vi "Color_Project.vi"() -> ()   [LabVIEW 2013]
uses:
  leitura de dados txt control.ctl
panel:
  out "Color Box":u32(colorbox)
  out "RGB":dbl[](array[numeric])
  in  "RGBStandards":string(combo)
  out "XYZ":dbl[](array[numeric])
  out "L*a*b*":dbl[](array[numeric])
  out "r1":dbl[](array[numeric])
  out "Reflectance2":string[][](array[string])
  out "teste":i32[](array[numeric])
  out "IL Table":string[][](array[string])
  out "ILCols":i32
  out "ILRows":i32
  out "Selected illuminant":dbl[](array[numeric])
  out "Reflectance":i32[](array[numeric])
  out "Is CMF selected?":bool
  out "Is illuminant selected?":bool
  out "Intepoled iluminants":dbl[][](array[numeric])
  out "Selected\nCMF":dbl[][](array[numeric])
  out "cmf Index":dbl
  out "CMFCols":i32
  out "CMFRows":i32
  out "CMF Table":string[][](array[string])
  in  "Color Matching Function":string(combo)
  out "Illuminant Graph":T1(graph)
  out "LambdaInterval":dbl[](array[numeric])
  out "NeedInterpolation?":bool
  out "Selected illuminant index":dbl
  in  "Select Illuminant":T2
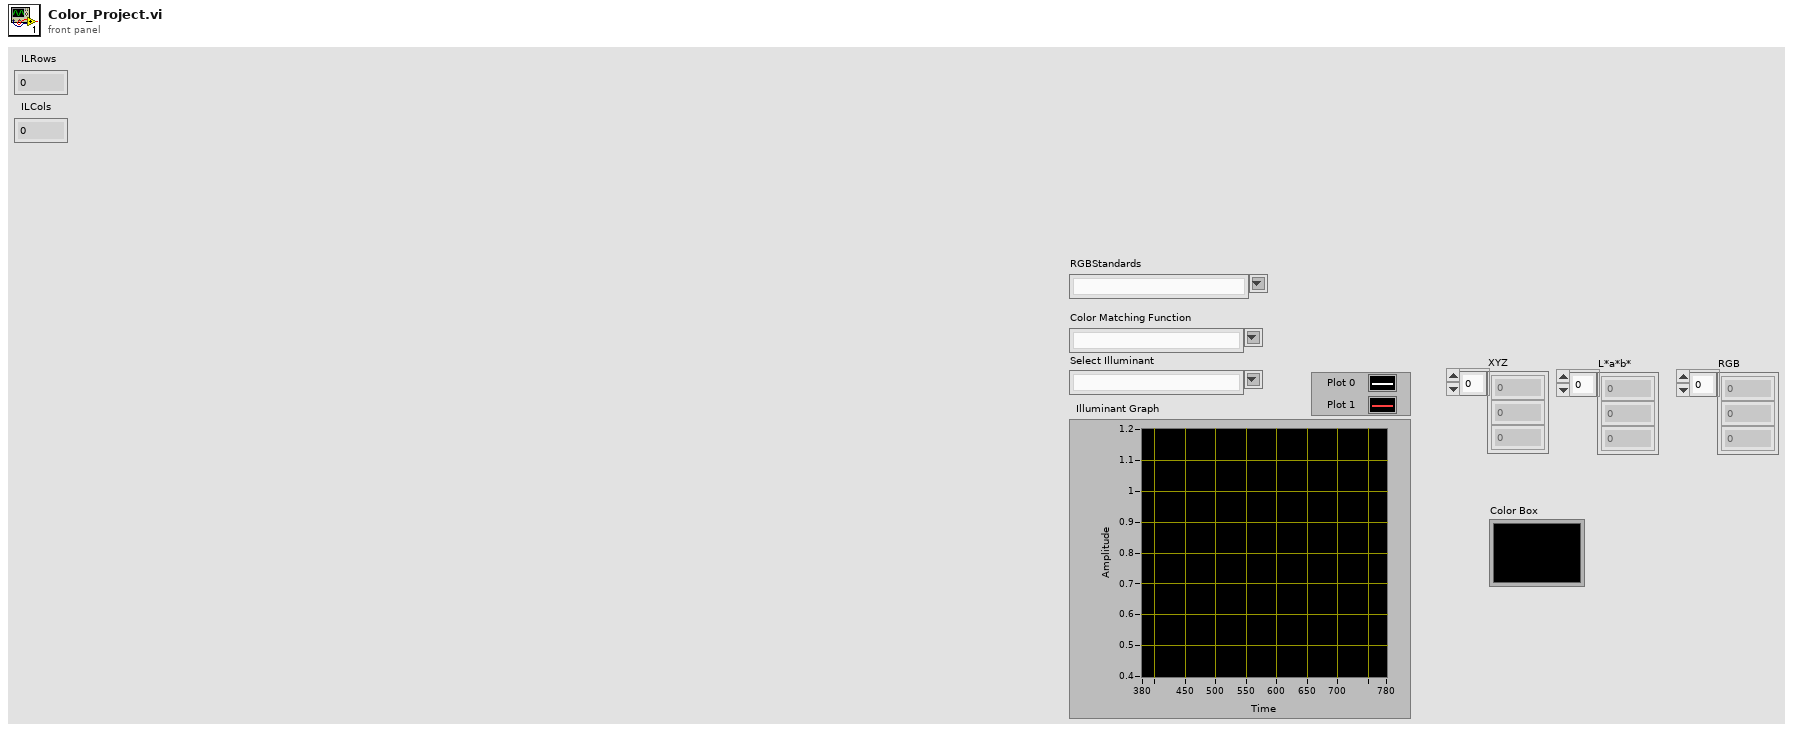
[diagram p1: front panel]
types:
  T1 = cluster{"GammaInterval":dbl[], "Interpolated":dbl[]}[]
  T2 = typedef "leitura de dados txt control.ctl" = string
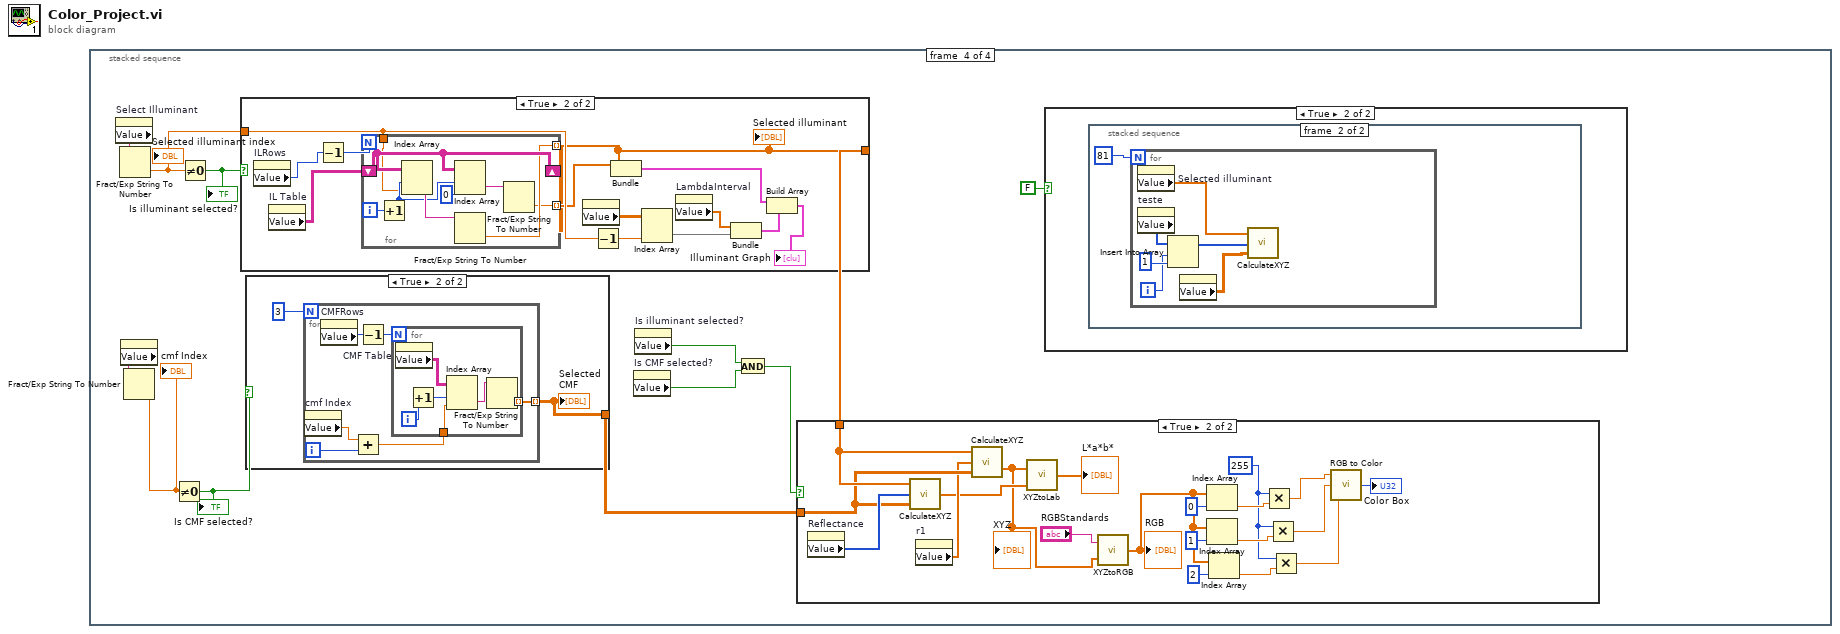
[diagram p0: block diagram]
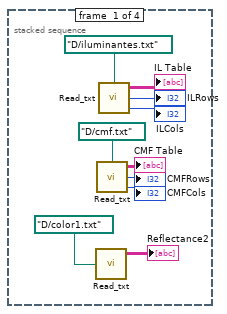
[diagram p2: hidden frame]
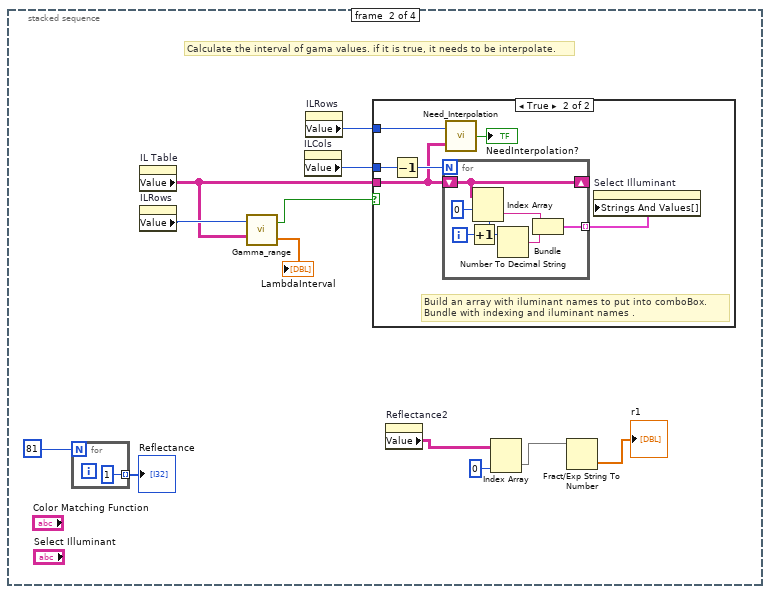
[diagram p3: hidden frame]
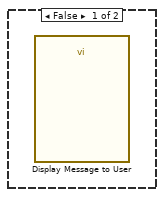
[diagram p4: hidden frame]
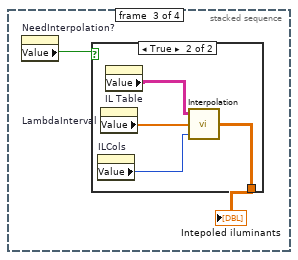
[diagram p5: hidden frame]
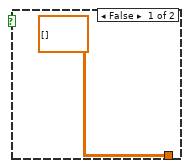
[diagram p6: hidden frame]
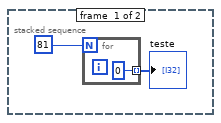
[diagram p8: hidden frame]
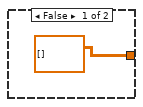
[diagram p10: hidden frame]
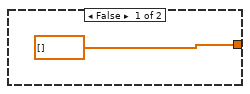
[diagram p11: hidden frame]
diagram:
  n1 = stacked-sequence {
    frame #0 {
      n2 = call "Read_txt.vi"("file path (dialog if empty)"=path "D:/color1.txt") -> ("Elements"=→"Reflectance2":string[][])  [unwired: 2 out]
      n3 = call "Read_txt.vi"("file path (dialog if empty)"=path "D:/cmf.txt") -> ("Elements"=→"CMF Table":string[][], "Rows"=→"CMFRows":i32, "Cols"=→"CMFCols":i32)
      n4 = call "Read_txt.vi"("file path (dialog if empty)"=path "D:/iluminantes.txt") -> ("Elements"=→"IL Table":string[][], "Rows"=→"ILRows":i32, "Cols"=→"ILCols":i32)
    }
    frame #1 {
      # "Calculate the interval of gama values. if it is true, it needs to be interpolate."
      n5 = for {
        N: 81 -> [_]
        tunnel: [1] -> w21 mode=indexing
      }
      "Reflectance" <- w21
      n6 = property on="IL Table" class="Arr (strict)"() -> ("Value"=w18:string[][])  [unwired: 2 in, 2 out]
      n7 = property on="ILRows" class="DigNum (strict)"() -> ("Value"=w19:i32)  [unwired: 2 in, 2 out]
      n8 = call "Gamma_range.vi"("Illuminant Table"=w18, "NumberOfRows"=w19) -> ("GammaInterval"=→"LambdaInterval":dbl[], "In range?"=w15:bool)
      n9 = property on="ILCols" class="DigNum (strict)"() -> ("Value"=w17:i32)  [unwired: 2 in, 2 out]
      n10 = property on="ILRows" class="DigNum (strict)"() -> ("Value"=w16:i32)  [unwired: 2 in, 2 out]
      n11 = case shown="True" w15 {
        tunnel: w18 -> [_ w24]
        tunnel: w17 -> [_ w25]
        tunnel: w16 -> [_ w23]
        frame False {
          n12 = call "Display Message to User"() -> ()  [unwired: 10 in, 2 out]
        }
        frame True {
          # "Build an array with iluminant names to put into comboBox.\nBundle with indexing and iluminant names ."
          n13 = Decrement(x=w25) -> (x-1=w27:i32)
          n14 = for {
            N: w27 -> [_]
            shift-right: [w33] -> _
            shift-left: w24 -> [w33]
            tunnel: [w29] -> w26 mode=indexing
            i -> [w35]
            n15 = Increment(x=w35) -> (x+1=w32:i32)
            n16 = Index Array(array=w33, index (row)=0, index (col)=w32) -> (element=w30:string)
            n17 = Number To Decimal String(number=w32) -> (decimal integer string=w31:string)  [unwired: 1 in]
            n18 = Bundle("String"=w30, w31) -> (w29:cluster{"String":string, string})  [unwired: 1 in]
          }
          n19 = call "Need_Interpolation.vi"("Matrix with txt"=w24, "Number of Rows"=w23) -> ("isNotFive?"=→"NeedInterpolation?":bool)
          n20 = property on="Select Illuminant" class="CmbBox (strict)"("Strings And Values[]"=w26) -> ()  [unwired: 2 in, 2 out]
        }
      }
      n21 = property on="Reflectance2" class="Arr (strict)"() -> ("Value"=w14:string[][])  [unwired: 2 in, 2 out]
      n22 = Index Array(array=w14, index (col)=0 ("disabled index (col)")) -> (element=w12:string[])  [unwired: 1 in]
      n23 = Fract/Exp String To Number(string=w12) -> (number=→"r1":dbl[])  [unwired: 3 in, 1 out]
    }
    frame #2 {
      n24 = property on="NeedInterpolation?" class="Bool (strict)"() -> ("Value"=w38:bool)  [unwired: 2 in, 2 out]
      n25 = case shown="True" w38 {
        tunnel: [dbl[][] [] w42] -> w37
        frame False {
        }
        frame True {
          n26 = property on="ILCols" class="DigNum (strict)"() -> ("Value"=w40:i32)  [unwired: 2 in, 2 out]
          n27 = property on="LambdaInterval" class="Arr (strict)"() -> ("Value"=w43:dbl[])  [unwired: 2 in, 2 out]
          n28 = property on="IL Table" class="Arr (strict)"() -> ("Value"=w41:string[][])  [unwired: 2 in, 2 out]
          n29 = call "Interpolation.vi"("Number of Columns"=w40, "Lambda Interval"=w43, "Illuminants"=w41) -> ("Interpolated"=w42:dbl[][])
        }
      }
      "Intepoled iluminants" <- w37
    }
    frame #3 {
      n30 = property on="Select Illuminant" class="CmbBox (strict)"() -> ("Value"=w51:T2)  [unwired: 2 in, 2 out]
      n31 = Fract/Exp String To Number(string=w51) -> (number=w50:dbl)  [unwired: 3 in, 1 out]
      "Selected illuminant index" <- w50
      n32 = property on="Color Matching Function" class="CmbBox"() -> ("Value"=w53:string)  [unwired: 2 in, 2 out]
      n33 = Fract/Exp String To Number(string=w53) -> (number=w54:dbl)  [unwired: 3 in, 1 out]
      "cmf Index" <- w54
      n34 = Not Equal To 0?(x=w54) -> (x != 0?=w52:bool)
      "Is CMF selected?" <- w52
      n35 = Not Equal To 0?(x=w50) -> (x != 0?=w55:bool)
      "Is illuminant selected?" <- w55
      n36 = case shown="True" w55 {
        tunnel: w50 -> [_ w110]
        tunnel: [dbl[] [] w104] -> w45
        frame False {
        }
        frame True {
          n37 = property on="ILRows" class="DigNum (strict)"() -> ("Value"=w103:i32)  [unwired: 2 in, 2 out]
          n38 = property on="IL Table" class="Arr (strict)"() -> ("Value"=w102:string[][])  [unwired: 2 in, 2 out]
          n39 = Decrement(x=w103) -> (x-1=w114:i32)
          n40 = for {
            N: w114 -> [_]
            shift-right: [w122] -> _
            shift-left: w102 -> [w122]
            tunnel: w110 -> [w115]
            tunnel: [w117] -> w104 mode=indexing
            tunnel: [w116] -> w106 mode=indexing
            i -> [w123]
            n41 = Increment(x=w123) -> (x+1=w118:i32)
            n42 = Index Array(array=w122, index (row)=w118, index (col)=w115) -> (element=w119:string)
            n43 = Index Array(array=w122, index (row)=w118, index (col)=0 ("disabled index (col)")) -> (element=w120:string)
            n44 = Fract/Exp String To Number(string=w119) -> (number=w117:dbl)  [unwired: 3 in, 1 out]
            n45 = Fract/Exp String To Number(string=w120) -> (number=w116:dbl)  [unwired: 3 in, 1 out]
          }
          "Selected illuminant" <- w104
          n46 = property on="Intepoled iluminants" class="Arr (strict)"() -> ("Value"=w108:dbl[][])  [unwired: 2 in, 2 out]
          n47 = Decrement(x=w110) -> (x-1=w109:dbl)
          n48 = Bundle(w106, w104) -> (w111:cluster{dbl[], dbl[]})  [unwired: 1 in]
          n49 = Index Array(array=w108, index (col)=w109) -> (element=w105:dbl[])  [unwired: 1 in]
          n50 = property on="LambdaInterval" class="Arr (strict)"() -> ("Value"=w107:dbl[])  [unwired: 2 in, 2 out]
          n51 = Bundle("Value"=w107, "Value"=w105) -> (w112:cluster{"Value":dbl[], "Value":dbl[]})  [unwired: 1 in]
          n52 = Build Array(w111, w112) -> (→"Illuminant Graph":cluster{"Value":dbl[], "Value":dbl[]}[])
        }
      }
      n53 = case shown="True" w52 {
        tunnel: [dbl[][] [] w87] -> w46
        frame False {
        }
        frame True {
          n54 = for {
            N: 3 -> [_]
            tunnel: [w91] -> w87 mode=indexing
            i -> [w93]
            n55 = property on="cmf Index" class="DigNum (strict)"() -> ("Value"=w94:dbl)  [unwired: 2 in, 2 out]
            n56 = property on="CMFRows" class="DigNum (strict)"() -> ("Value"=w90:i32)  [unwired: 2 in, 2 out]
            n57 = Add(x=w94, y=w93) -> (x+y=w92:dbl)
            n58 = Decrement(x=w90) -> (x-1=w89:i32)
            n59 = for {
              N: w89 -> [_]
              tunnel: w92 -> [w99]
              tunnel: [w95] -> w91 mode=indexing
              i -> [w98]
              n60 = property on="CMF Table" class="Arr (strict)"() -> ("Value"=w100:string[][])  [unwired: 2 in, 2 out]
              n61 = Increment(x=w98) -> (x+1=w97:i32)
              n62 = Index Array(array=w100, index (row)=w97, index (col)=w99) -> (element=w96:string)
              n63 = Fract/Exp String To Number(string=w96) -> (number=w95:dbl)  [unwired: 3 in, 1 out]
            }
          }
          "Selected\nCMF" <- w87
        }
      }
      n64 = property on="Is CMF selected?" class="Bool (strict)"() -> ("Value"=w48:bool)  [unwired: 2 in, 2 out]
      n65 = property on="Is illuminant selected?" class="Bool (strict)"() -> ("Value"=w49:bool)  [unwired: 2 in, 2 out]
      n66 = And(x=w49, y=w48) -> (x .and. y?=w47:bool)
      n67 = case shown="True" w47 {
        tunnel: w45 -> [_ w84]
        tunnel: w46 -> [_ w83]
        frame False {
        }
        frame True {
          w69 = 255
          n68 = property on="Reflectance" class="Arr (strict)"() -> ("Value"=w85:i32[])  [unwired: 2 in, 2 out]
          n69 = call "CalculateXYZ.vi"("CMF"=w83, "Reflectance"=w85, "Illuminant"=w84) -> ("XYZ"=w81:dbl[])
          n70 = property on="r1" class="Arr (strict)"() -> ("Value"=w82:dbl[])  [unwired: 2 in, 2 out]
          n71 = call "CalculateXYZ.vi"("CMF"=w83, "Reflectance"=w82, "Illuminant"=w84) -> ("XYZ"=w79:dbl[])
          "XYZ" <- w79
          n72 = call "XYZtoLab.vi"("XrYrZr"=w81, "XYZ"=w79) -> ("L*a*b*"=→"L*a*b*":dbl[])
          n73 = call "XYZtoRGB.vi"("XYZ"=w79, "RGBStandards"="RGBStandards") -> ("RGB"=w76:dbl[])
          "RGB" <- w76
          n74 = Index Array(array=w76, index=0) -> (element=w72:dbl)
          n75 = Index Array(array=w76, index=1) -> (element=w70:dbl)
          n76 = Index Array(array=w76, index=2) -> (element=w71:dbl)
          n77 = Multiply(x=w69, y=w72) -> (x*y=w68:dbl)
          n78 = Multiply(x=w69, y=w70) -> (x*y=w67:dbl)
          n79 = Multiply(x=w69, y=w71) -> (x*y=w66:dbl)
          n80 = call <vilib>:"RGB to Color.vi"("B"=w66, "G"=w67, "R"=w68) -> ("Color"=→"Color Box":u32)
        }
      }
      n81 = case shown="True" FALSE {
        frame False {
        }
        frame True {
          n82 = stacked-sequence {
            frame #0 {
              n83 = for {
                N: 81 -> [_]
                tunnel: [0] -> w56 mode=indexing
              }
              "teste" <- w56
            }
            frame #1 {
              n84 = for {
                N: 81 -> [_]
                i -> [w64]
                n85 = property on="Selected illuminant" class="Arr (strict)"() -> ("Value"=w62:dbl[])  [unwired: 2 in, 2 out]
                n86 = property on="teste" class="Arr (strict)"() -> ("Value"=w63:i32[])  [unwired: 2 in, 2 out]
                n87 = Insert Into Array(array=w63, index=w64, new element=1 ("new element/subarray")) -> (w61:i32[])
                n88 = property on="Selected\nCMF" class="Arr (strict)"() -> ("Value"=w60:dbl[][])  [unwired: 2 in, 2 out]
                n89 = call "CalculateXYZ.vi"("CMF"=w60, "Reflectance"=w61, "Illuminant"=w62) -> ()  [unwired: 1 out]
              }
            }
          }
        }
      }
    }
  }
